vi "Descriptor_GetFromVariant.vi"(10 "Variant":variant) -> (1 "name":string, 2 "Descriptor":T1)   [LabVIEW 2013, in "OpenDescriptor.lvlib"]
uses:
  OpenDescriptor.lvlib
  OpenDescriptor -- cluster.ctl
  TypeDescriptor_GetPString.vi
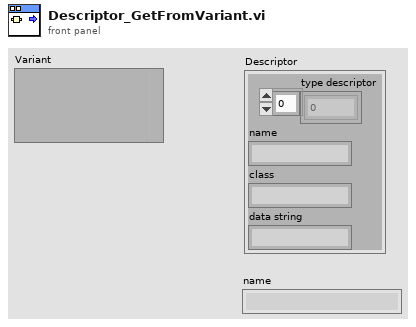
[diagram p1: front panel]
types:
  T1 = typedef "OpenDescriptor.lvlib/OpenDescriptor -- cluster.ctl" = cluster{"type descriptor":i16[], "name":string, "class":string, "data string":string}
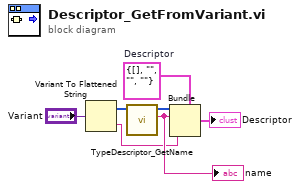
[diagram p0: block diagram]
diagram:
  w7 = T1 {"type descriptor"=[], "name"="", "class"="", "data string"=""}  # Descriptor
  n1 = Variant To Flattened String(Variant="Variant") -> (data string=w3:string, 1:w6:i16[])
  n2 = call "TypeDescriptor_GetName.vi"("type descriptor"=w6) -> ("name"=w4:string, "type descriptor dup"=w5:i16[])  [unwired: 8 in, 1 out]
  "name" <- w4
  n3 = Bundle(cluster=w7, "type descriptor"=w5, "name"=w4, "data string"=w3) -> (→"Descriptor":T1)  [unwired: 1 in]
